vi "CHP Servo SG Power.vi"(0 "SA Resource":refnum<k21>, 5 "RFSG Handle":refnum<k15>, 7 "Power Servo Settings":T3={"Desired TxP Power (dBm)"=0.0, "Tolerance (dB)"=0.05, "Max Number of Iterations"=0, "AutoLevel Settings"={"Reference Level"=30.0, "Auto-Level Reference Level"=FALSE, "Auto-Level Measurement Time"=0.01, "Auto-Level Bandwidth"=0.01}} {"AutoLevel Settings"."Auto-Level Bandwidth" format="%#_6p"; "AutoLevel Settings"."Auto-Level Measurement Time" format="%#_6p"; "AutoLevel Settings"."Reference Level" format="%#_6p"}, 11 "error in (no error)":errorcluster) -> (4 "SA Resource Out":T1, 6 "CHP Servo Results":T2, 15 "error Out":errorcluster)   [LabVIEW 2016, in "RFmxSpecAn.lvlib"]
uses:
  RFmxSpecAn.lvlib
  <vilib>/RFmx/SpecAn/mx/RFmxSpecAn.llb/RFmxSpecAn Select Measurement (Single).vi
  <vilib>/RFmx/SpecAn/mx/RFmxSpecAn.llb/RFmxSpecAn CHP Fetch Total Carrier Power.vi
  <vilib>/RFmx/SpecAn/mx/RFmxSpecAn.llb/RFmxSpecAn CHP Fetch Spectrum.vi
  Typedefs/CHP Servo Results.ctl
  Typedefs/AutoLevel Settings.ctl
  Typedefs/CHP Power Servo Settings.ctl
  <vilib>/RFmx/RFInstr/mx/Support/RFmxInstrSupport.llb/niRFmx Instrument Handle.ctl
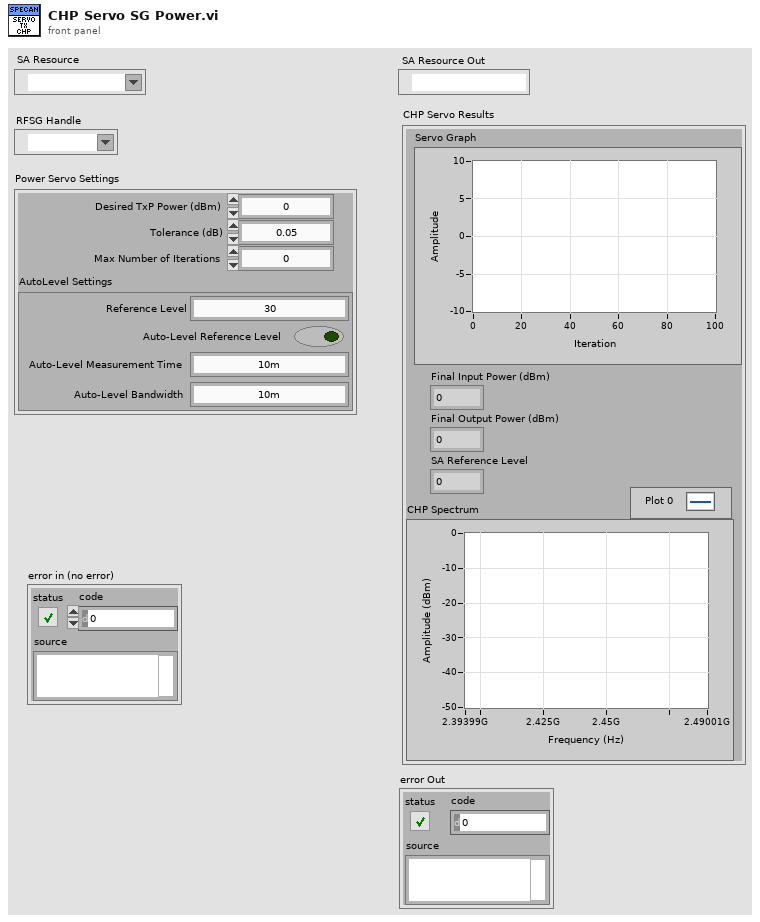
[diagram p1: front panel]
types:
  T1 = typedef "niRFmx Instrument Handle.ctl" = refnum<k21>
  T2 = typedef "RFmxSpecAn.lvlib/CHP Servo Results.ctl" = cluster{"Servo Graph":dbl[], "Final Input Power (dBm)":dbl, "SA Reference Level":dbl, "Final Output Power (dBm)":dbl, "CHP Spectrum":cluster{"x0":dbl, "dx":dbl, "y":sgl[]}}
  T3 = typedef "RFmxSpecAn.lvlib/CHP Power Servo Settings.ctl" = cluster{"Desired TxP Power (dBm)":dbl, "Tolerance (dB)":dbl, "Max Number of Iterations":i32, "AutoLevel Settings":T4}
  T4 = typedef "RFmxSpecAn.lvlib/AutoLevel Settings.ctl" = cluster{"Reference Level":dbl, "Auto-Level Reference Level":bool, "Auto-Level Measurement Time":dbl, "Auto-Level Bandwidth":dbl}
  T5 = enum16{"ACP", "CCDF", "CHP", "FCnt", "Harmonics", "OBW", "SEM", "Spectrum", "Spur", "TXP", "AMPM", "DPD", "IQ", "IM", "NF", "PhaseNoise"}
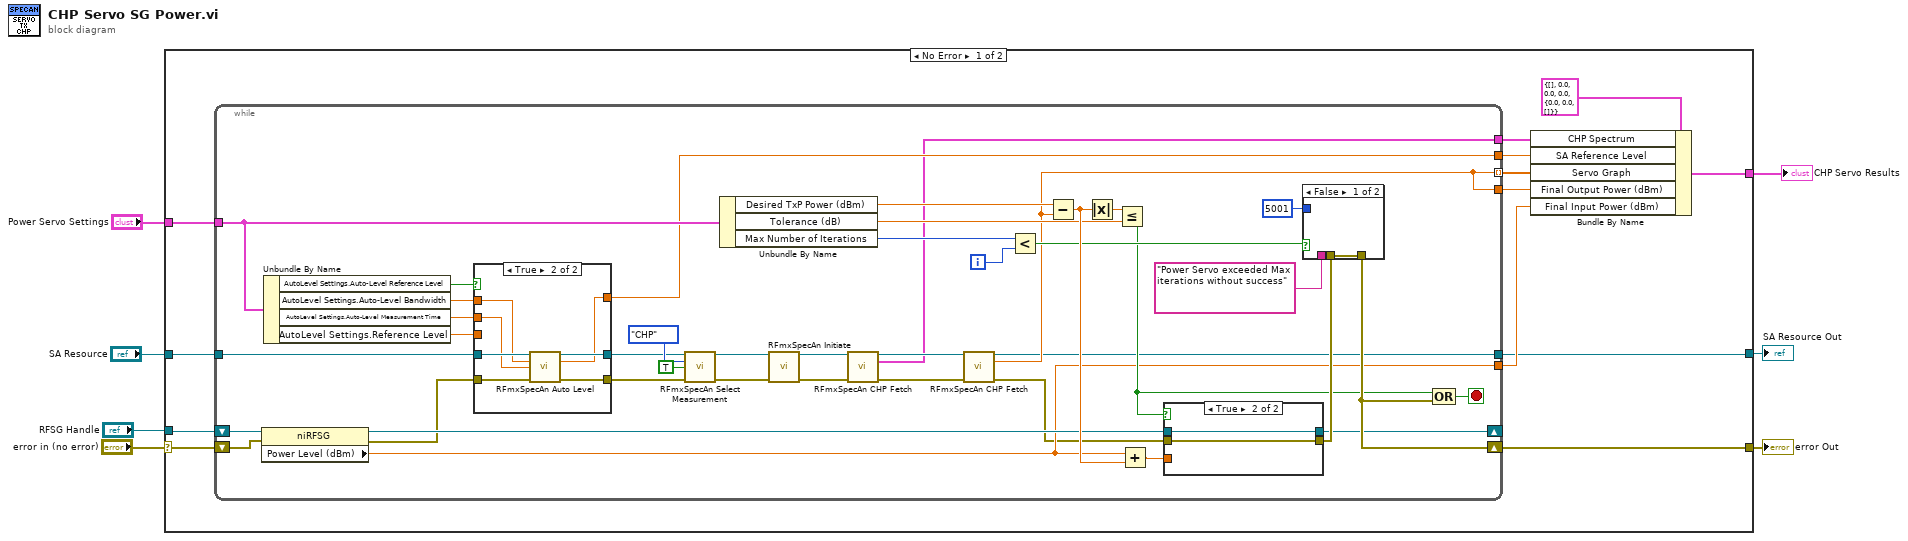
[diagram p0: block diagram]
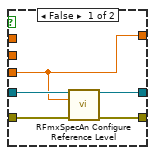
[diagram p2: hidden frame]
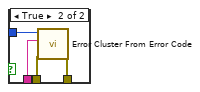
[diagram p3: hidden frame]
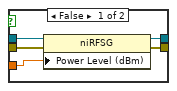
[diagram p4: hidden frame]
diagram:
  n1 = case shown="No Error" "error in (no error)" {
    selector: "error in (no error)" -> [w20 w87]
    tunnel: "RFSG Handle" -> [w19 _]
    tunnel: "Power Servo Settings" -> [w18 _]
    tunnel: "SA Resource" -> [w17 w86]
    tunnel: [w11 _] -> w3
    tunnel: [w10 w87] -> w2
    tunnel: [w9 w86] -> w1
    frame No Error {
      n2 = while {
        shift-right: [w42] -> w10
        shift-left: w20 -> [w60]
        shift-right: [w28] -> _
        shift-left: w19 -> [w61]
        tunnel: w18 -> [w52]
        tunnel: w17 -> [w36]
        tunnel: [w40] -> w12
        tunnel: [w29] -> w14 mode=indexing
        tunnel: [w30] -> w15
        tunnel: [w29] -> w13
        tunnel: [w27] -> w9
        tunnel: [w22] -> w8
        i -> [w48]
        stop <- w43 stop-if-true
        n3 = property class="niRFSG"(reference=w61, error in=w60) -> (reference out=w53:refnum<k15>, error out=w33:errorcluster, "Power Level (dBm)"=w40:dbl)
        n4 = Unbundle By Name(w52) -> ("AutoLevel Settings.Auto-Level Reference Level"=w38:bool, "AutoLevel Settings.Auto-Level Bandwidth"=w37:dbl, "AutoLevel Settings.Auto-Level Measurement Time"=w31:dbl, "AutoLevel Settings.Reference Level"=w32:dbl)
        n5 = case shown="True" w38 {
          tunnel: w37 -> [_ w68]
          tunnel: w36 -> [w66 w73]
          tunnel: [w63 w72] -> w35
          tunnel: [w64 w71] -> w34
          tunnel: w33 -> [w65 w70]
          tunnel: w32 -> [w62 _]
          tunnel: w31 -> [_ w69]
          tunnel: [w62 w67] -> w30
          frame False {
            n6 = call <vilib>:"RFmxSpecAn Configure Reference Level.vi"("Instrument Handle In"=w66, "Reference Level"=w62, "error in (no error)"=w65) -> ("Instrument Handle Out"=w63:refnum<k21>, "error out"=w64:errorcluster)  [unwired: 11 in]
          }
          frame True {
            n7 = call <vilib>:"RFmxSpecAn Auto Level.vi"("Instrument Handle In"=w73, "Bandwidth (Hz)"=w68, "Measurement Interval (s)"=w69, "error in (no error)"=w70) -> ("Instrument Handle Out"=w72:refnum<k21>, "Reference Level"=w67:dbl, "error out"=w71:errorcluster)  [unwired: 9 in]
          }
        }
        n8 = call-poly <vilib>:"RFmxSpecAn Select Measurement.vi"("Instrument Handle In"=w35, "Measurement"=T5."CHP", "Enable All Traces"=TRUE, "error in (no error)"=w34) -> ("Instrument Handle Out"=w50:refnum<k21>, "error out"=w51:errorcluster)  [unwired: 10 in]
        n9 = Unbundle By Name(w52) -> ("Desired TxP Power (dBm)"=w57:dbl, "Tolerance (dB)"=w55:dbl, "Max Number of Iterations"=w56:i32)
        n10 = call <vilib>:"RFmxSpecAn Initiate.vi"("Instrument Handle In"=w50, "error in (no error)"=w51) -> ("Instrument Handle Out"=w26:refnum<k21>, "error out"=w24:errorcluster)  [unwired: 11 in, 1 out]
        n11 = call-poly <vilib>:"RFmxSpecAn CHP Fetch.vi"("Instrument Handle In"=w26, "error in (no error)"=w24) -> ("Instrument Handle Out"=w25:refnum<k21>, "Spectrum (dBm)"=w22:cluster{"x0":dbl, "dx":dbl, "y":sgl[]}, "error out"=w23:errorcluster)  [unwired: 11 in]
        n12 = call-poly <vilib>:"RFmxSpecAn CHP Fetch.vi"("Instrument Handle In"=w25, "error in (no error)"=w23) -> ("Instrument Handle Out"=w27:refnum<k21>, "Total Carrier Power (dBm)"=w29:dbl, "error out"=w39:errorcluster)  [unwired: 11 in]
        n13 = Less?(x=w56, y=w48) -> (x < y?=w44:bool)
        n14 = Subtract(x=w57, y=w29) -> (x-y=w58:dbl)
        n15 = Absolute Value(x=w58) -> (abs(x)=w54:dbl)
        n16 = Less Or Equal?(x=w54, y=w55) -> (x <= y?=w41:bool)
        n17 = Add(x=w40, y=w58) -> (x+y=w59:dbl)
        n18 = case shown="True" w41 {
          tunnel: w53 -> [w83 w84]
          tunnel: w59 -> [w82 _]
          tunnel: w39 -> [w81 w85]
          tunnel: [w80 w85] -> w46
          tunnel: [w79 w84] -> w28
          frame False {
            n19 = property class="niRFSG"(reference=w83, error in=w81, "Power Level (dBm)"=w82) -> (reference out=w79:refnum<k15>, error out=w80:errorcluster)
          }
          frame True {
          }
        }
        n20 = case shown="False" w44 {
          tunnel: w46 -> [w74 w78]
          tunnel: [w74 w77] -> w42
          tunnel: "Power Servo exceeded Max iterations without success" ("error message (\"\")") -> [_ w76]
          tunnel: 5001 ("code") -> [_ w75]
          frame False {
          }
          frame True {
            n21 = call <vilib>:"Error Cluster From Error Code.vi"("error in (no error)"=w78, "error message (\"\")"=w76, "error code (0)"=w75) -> ("error out"=w77:errorcluster)  [unwired: 6 in]
          }
        }
        n22 = Compound Arithmetic op=OR(w41, w42) -> (w43:bool)
      }
      n23 = Bundle By Name(cluster=T2 {"Servo Graph"=[], "Final Input Power (dBm)"=0.0, "SA Reference Level"=0.0, "Final Output Power (dBm)"=0.0, "CHP Spectrum"={"x0"=0.0, "dx"=0.0, "y"=[]}} ("TXP Servo Results"), "CHP Spectrum"=w8, "SA Reference Level"=w15, "Servo Graph"=w14, "Final Output Power (dBm)"=w13, "Final Input Power (dBm)"=w12) -> (w11:T2)
    }
    frame Error {
    }
  }
  "CHP Servo Results" <- w3
  "error Out" <- w2
  "SA Resource Out" <- w1
